vi "dec_wrap-around.vi"(7 "DEC IN (°)":dbl format="%.8f") -> (8 "DEC OUT (°)":dbl format="%.8f")   [LabVIEW 2019]
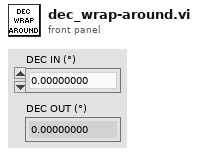
[diagram p1: front panel]
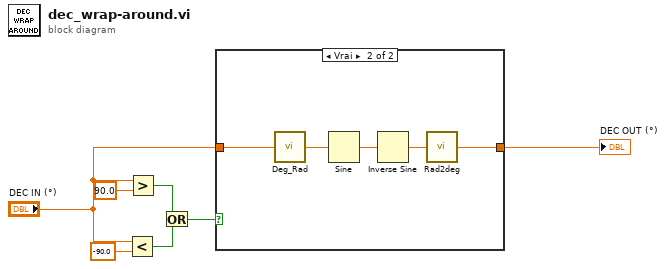
[diagram p0: block diagram]
diagram:
  n1 = Less?(x="DEC IN (°)", y=-90.0) -> (x < y?=w4:bool)
  n2 = Greater?(x="DEC IN (°)", y=90.0) -> (0:w5:bool)
  n3 = Or(x=w5, y=w4) -> (x .or. y?=w3:bool)
  n4 = case shown="Vrai" w3 {
    tunnel: "DEC IN (°)" -> [w8 w13]
    tunnel: [w8 w9] -> w1
    frame False {
    }
    frame True {
      n5 = call "Deg_Rad.vi"("Angle"=w13) -> ("RadRot"=w12:dbl)
      n6 = Sine(x=w12) -> (sin(x)=w11:dbl)
      n7 = Inverse Sine(1:w11) -> (0:w10:dbl)
      n8 = call "Rad2deg.vi"("rad"=w10) -> ("deg"=w9:dbl)
    }
  }
  "DEC OUT (°)" <- w1
